vi "VI_UpdateXYGraphData.vi"(8 "error in (no error)":errorcluster, 10 "Old Graph Data":T1[](array[typedef]), 11 "Common Refs":T2={"LBox_ChList"=refnum, "STR_LoggingChName1"=refnum, "Listbox_ChValue"=refnum, "STR_LoggingChName2"=refnum, "STR_LoggingChName3"=refnum, "STR_LoggingChName4"=refnum, "STR_LoggingChName5"=refnum, "STR_LoggingChName6"=refnum, "OXY_SCPI Ref"="TCPIP0::192.168.1.75::10001::SOCKET", "STR_ChName1"=refnum, "STR_ChName2"=refnum, "STR_ChName3"=refnum, "STR_ChName4"=refnum, "STR_ChName5"=refnum, "STR_ChName6"=refnum, "Enum_SelectTimestampFormat"=refnum, "GRAPH-XY_ELOG"=refnum, "GRAPH-XY_Measurement"=refnum, "Button_StartBuffer"=refnum, "Button_StopBuffer"=refnum, "Button_FetchData"=refnum, "STR_LoggingChName1"=refnum, "STR_LoggingChName2"=refnum, "STR_LoggingChName3"=refnum, "STR_LoggingChName4"=refnum, "STR_LoggingChName5"=refnum, "STR_LoggingChName6"=refnum, "Enum_SelectCalc"=refnum, "Num_SetDurationTime"=refnum, "Button_StopTransfer"=refnum, "Button_StartTransfer"=refnum, "STR_IN_AggregationRate"=refnum, "Button_Disconnect"=refnum, "Button_Connect"=refnum, "Button_StartRec"=refnum, "Button_PauseRec"=refnum, "Button_StopRec"=refnum, "Bool_StatusLED"=refnum, "Indicator_RecordingStatus"=refnum}) -> (0 "error out":errorcluster, 1 "Latest Value per Item":dbl[](array[numeric]), 2 "Updated Graph Data":T1[](array[typedef]))   [LabVIEW 2018]
uses:
  TypeDefs/Graph_DataArrayElement.ctl
  TypeDefs/Refs_Common.ctl
  OXYGEN/VIs/Measurement Values/SubVIs/MeasurementItems_GetChannelDimension.vi
  OXYGEN.lvlib
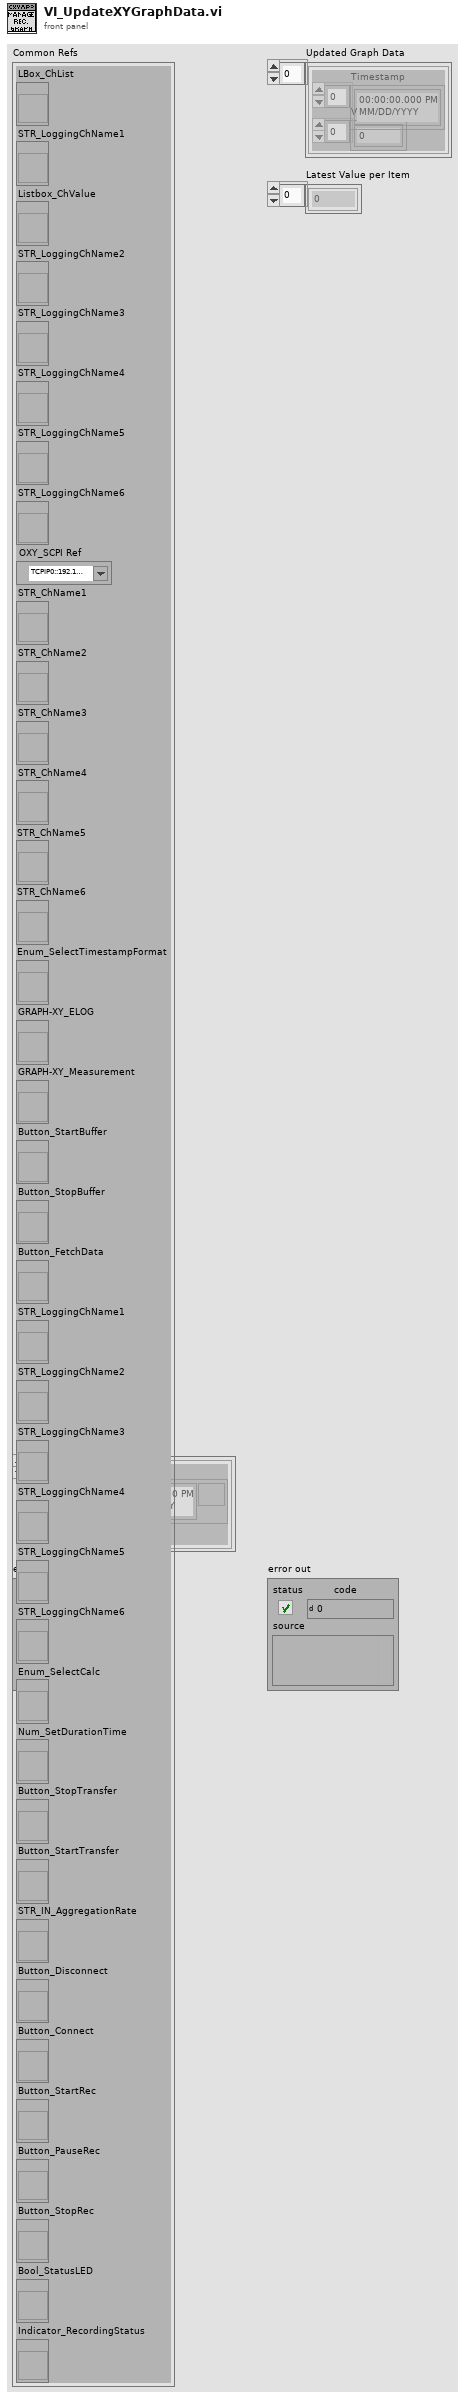
[diagram p1: front panel]
types:
  T1 = typedef "Graph_DataArrayElement.ctl" = cluster{"Timestamp":timestamp[], "Value":dbl[]}
  T2 = typedef "Refs_Common.ctl" = cluster{"LBox_ChList":refnum<vi>, "STR_LoggingChName1":refnum<vi>, "Listbox_ChValue":refnum<vi>, "STR_LoggingChName2":refnum<vi>, "STR_LoggingChName3":refnum<vi>, "STR_LoggingChName4":refnum<vi>, "STR_LoggingChName5":refnum<vi>, "STR_LoggingChName6":refnum<vi>, "OXY_SCPI Ref":refnum<visa-resource-name>, "STR_ChName1":refnum<vi>, "STR_ChName2":refnum<vi>, "STR_ChName3":refnum<vi>, "STR_ChName4":refnum<vi>, "STR_ChName5":refnum<vi>, "STR_ChName6":refnum<vi>, "Enum_SelectTimestampFormat":refnum<vi>, "GRAPH-XY_ELOG":refnum<vi>, "GRAPH-XY_Measurement":refnum<vi>, "Button_StartBuffer":refnum<vi>, "Button_StopBuffer":refnum<vi>, "Button_FetchData":refnum<vi>, "STR_LoggingChName1":refnum<vi>, "STR_LoggingChName2":refnum<vi>, "STR_LoggingChName3":refnum<vi>, "STR_LoggingChName4":refnum<vi>, "STR_LoggingChName5":refnum<vi>, "STR_LoggingChName6":refnum<vi>, "Enum_SelectCalc":refnum<vi>, "Num_SetDurationTime":refnum<vi>, "Button_StopTransfer":refnum<vi>, "Button_StartTransfer":refnum<vi>, "STR_IN_AggregationRate":refnum<vi>, "Button_Disconnect":refnum<vi>, "Button_Connect":refnum<vi>, "Button_StartRec":refnum<vi>, "Button_PauseRec":refnum<vi>, "Button_StopRec":refnum<vi>, "Bool_StatusLED":refnum<vi>, "Indicator_RecordingStatus":refnum<vi>}
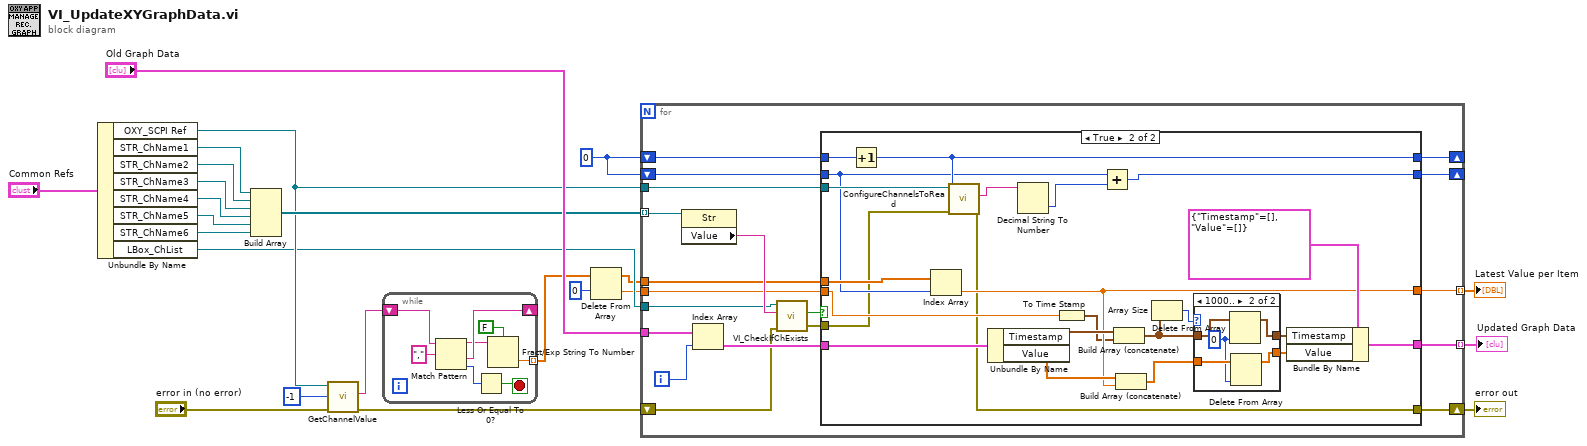
[diagram p0: block diagram]
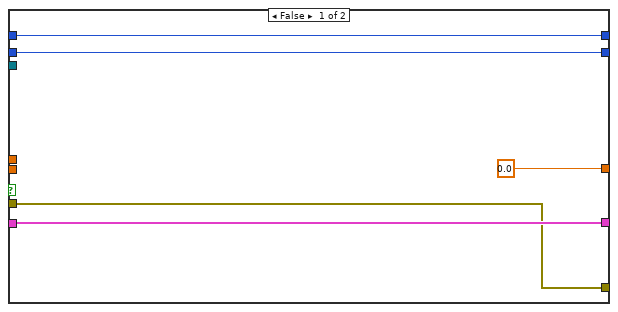
[diagram p2: hidden frame]
diagram:
  w10 = i64 0 ("Channel (-1 for all)")
  n1 = Unbundle By Name("Common Refs") -> ("OXY_SCPI Ref"=w11:refnum<visa-resource-name>, "STR_ChName1"=w20:refnum<vi>, "STR_ChName2"=w19:refnum<vi>, "STR_ChName3"=w18:refnum<vi>, "STR_ChName4"=w17:refnum<vi>, "STR_ChName5"=w16:refnum<vi>, "STR_ChName6"=w15:refnum<vi>, "LBox_ChList"=w9:refnum<vi>)
  n2 = Build Array(w20, w19, w18, w17, w16, w15) -> (w14:refnum<vi>[])
  n3 = call "GetChannelValue.vi"("error in (no error)"="error in (no error)", "#Channel (-1 fo all)"=i64 -1 ("Channel (-1 for all)"), "OXY_SCPI Reseource In"=w11) -> ("error out"=w3:errorcluster, "Value List"=w2:string)  [unwired: 5 in, 2 out]
  n4 = while {
    shift-right: [w29] -> _
    shift-left: w2 -> [w31]
    tunnel: [w24] -> w1 mode=indexing
    stop <- w26 stop-if-true
    n5 = Match Pattern(string=w31, regular expression=",") -> (before substring=w28:string, after substring=w29:string, offset past match=w25:i32)  [unwired: 1 in, 1 out]
    n6 = Less Or Equal To 0?(x=w25) -> (x <= 0?=w26:bool)
    n7 = Fract/Exp String To Number(use system decimal point (T)=FALSE, string=w28) -> (number=w24:dbl)  [unwired: 2 in, 1 out]
  }
  n8 = Delete From Array(array=w1, index=0) -> (deleted portion=w6:dbl, array with subset deleted=w7:dbl[])  [unwired: 1 in]
  n9 = for {
    tunnel: "Old Graph Data" -> [w49]
    tunnel: [w50] -> w22 mode=indexing
    tunnel: w14 -> [w46] mode=indexing
    shift-right: [w42] -> w13
    shift-left: w3 -> [w44]
    shift-right: [w39] -> _
    shift-left: w10 -> [w40]
    tunnel: w7 -> [w38]
    tunnel: w11 -> [w37]
    shift-right: [w35] -> _
    shift-left: w10 -> [w36]
    tunnel: w9 -> [w34]
    tunnel: w6 -> [w33]
    tunnel: [w32] -> w5 mode=indexing
    i -> [w48]
    n10 = property class="Str"(reference=w46) -> ("Value"=w41:string)  [unwired: 1 in, 2 out]
    n11 = Index Array(array=w49, index=w48) -> (element=w47:T1)
    n12 = call "VI_CheckIfChExists.vi"("error in (no error)"=w44, "Channel Name To Check"=w41, "ChList_Ref In"=w34) -> ("error out"=w45:errorcluster, "Channel Exists"=w43:bool)  [unwired: 6 in, 1 out]
    n13 = case shown="True" w43 {
      tunnel: [w54 w78] -> w32
      tunnel: [0.0 ("Value") w72] -> w50
      tunnel: w47 -> [w54 w77]
      tunnel: w45 -> [w53 w57]
      tunnel: [w53 w56] -> w42
      tunnel: w40 -> [w52 w70]
      tunnel: [w52 w69] -> w39
      tunnel: w38 -> [_ w73]
      tunnel: w37 -> [_ w71]
      tunnel: w36 -> [w51 w65]
      tunnel: [w51 w66] -> w35
      tunnel: w33 -> [_ w64]
      frame False {
      }
      frame True {
        n14 = Increment(x=w70) -> (x+1=w69:i64)
        n15 = Index Array(array=w73, index=w65) -> (element=w72:dbl)
        n16 = call-poly "ConfigureChannelsToRead.vi"("error in (no error)"=w57, "#Channel"=w69, "OXY_SCPI Reseource In"=w71) -> ("error out"=w56:errorcluster, "Range"=w68:string)  [unwired: 5 in, 2 out]
        n17 = Unbundle By Name(w77) -> ("Timestamp"=w74:timestamp[], "Value"=w75:dbl[])
        n18 = Decimal String To Number(string=w68) -> (number=w67:i32)  [unwired: 2 in, 1 out]
        n19 = To Time Stamp(1:w64) -> (0:w63:timestamp)
        n20 = Add(x=w65, y=w67) -> (x+y=w66:i64)
        n21 = Build Array (concatenate)(w74, w63) -> (w61:timestamp[])
        n22 = Build Array (concatenate)(w75, w72) -> (w60:dbl[])
        n23 = Array Size(array=w61) -> (size(s)=w62:i32)
        n24 = case shown="1000.." w62 {
          tunnel: w61 -> [w80 w85]
          tunnel: w60 -> [w79 w84]
          tunnel: [w79 w83] -> w59
          tunnel: [w80 w82] -> w58
          frame Default {
          }
          frame 1000.. {
            w81 = 0 ("index")
            n25 = Delete From Array(array=w85, index=w81) -> (array with subset deleted=w82:timestamp[])  [unwired: 1 in, 1 out]
            n26 = Delete From Array(array=w84, index=w81) -> (array with subset deleted=w83:dbl[])  [unwired: 1 in, 1 out]
          }
        }
        n27 = Bundle By Name(cluster=T1 {"Timestamp"=[], "Value"=[]} ("Data Element"), "Timestamp"=w58, "Value"=w59) -> (w78:T1)
      }
    }
  }
  "error out" <- w13
  "Latest Value per Item" <- w22
  "Updated Graph Data" <- w5
